vi "Get Parameter Value - Array of Strings.vi"(7 "Default value":string[](array[string]), 8 "error in (no error)":errorcluster, 9 "Parameter name":string, 10 "Config name":string, 11 "Config in":refnum<class "Config.lvclass">) -> (0 "error out":errorcluster, 2 "Value":string[](array[string]), 3 "Config out":refnum<class "Config.lvclass">)   [LabVIEW 2026, in "TALOS.lvlib" / "Classes.lvlib" / "Config.lvclass"]
doc: "Get the parameter's value (string) from the specified configuration. Use the data type terminal to specify the output type."
uses:
  Config.lvclass
  <vilib>/AdvancedString/Delimited String to 1D String Array (string).vi
  <vilib>/Utility/error.llb/Trim Whitespace (string).vi
  <vilib>/Utility/error.llb/Trim Whitespace One-Sided.vi
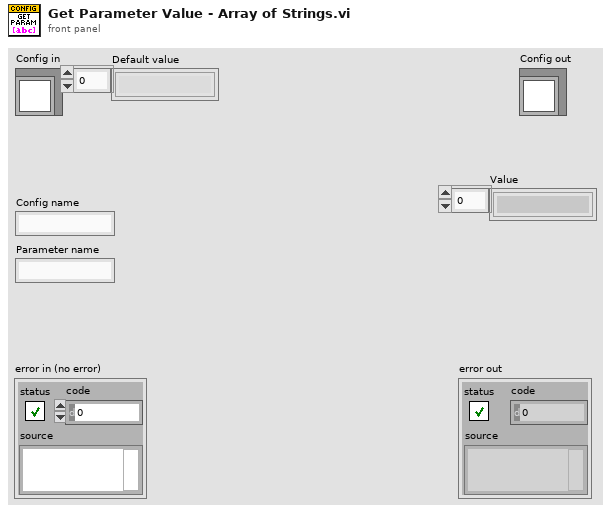
[diagram p1: front panel]
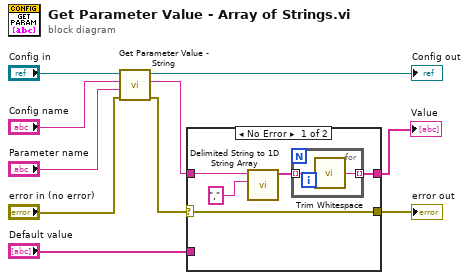
[diagram p0: block diagram]
diagram:
  n1 = call "Get Parameter Value - String.vi"("error in (no error)"="error in (no error)", "Parameter name"="Parameter name", "Config name"="Config name", "Config in"="Config in") -> ("error out"=w5:errorcluster, "Value"=w4:string, "Config out"=→"Config out":refnum<class "Config.lvclass">)  [unwired: 5 in]
  n2 = case shown="No Error" w5 {
    selector: w5 -> [w12 w18]
    tunnel: w4 -> [w15 _]
    tunnel: "Default value" -> [_ w19]
    tunnel: [w12 w18] -> w1
    tunnel: [w11 w19] -> w3
    frame No Error {
      n3 = call-poly <vilib>:"Delimited String to 1D String Array.vi"("delimiter"=",", "delimited string"=w15) -> ("string array"=w13:string[])  [unwired: 9 in]
      n4 = for {
        tunnel: w13 -> [w17] mode=indexing
        tunnel: [w16] -> w11 mode=indexing
        n5 = call-poly <vilib>:"Trim Whitespace.vi"("string"=w17) -> ("trimmed string"=w16:string)  [unwired: 1 in]
      }
    }
    frame Error {
    }
  }
  "error out" <- w1
  "Value" <- w3
